vi "XIPIN_Video_In_to_AXI4-Stream_4_0.vi"   [LabVIEW 2017]
doc: "Video bridge converting native video to AXI4-Stream.\n------------------------------------\n<b>Need License</b> : No\n<b>Interface</b> : AXI4-Stream"
uses:
  <vilib>/rvi/XilinxIP/XIPIN_XNode/niFpgaXIPIN.xnode
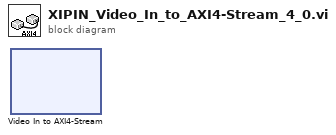
[diagram p0: block diagram]
diagram:
  n1 = xnode ("Video In to AXI4-Stream")() -> ()
